vi "Test Analysis Module.vi"() -> ()   [LabVIEW 2013]
uses:
  <vilib>/rvi/Emulation/niFpgaSctlEmulationGetInTimedLoop.vi
  <vilib>/rvi/Emulation/niFpgaEmulationReportErrorSimple.vi
  <vilib>/rvi/Emulation/niFpgaGetClockAttributes.vi
  <vilib>/rvi/Emulation/niFpgaCriticalErrorInLSC.vi
  <vilib>/rvi/FIFO/Fifo_Resource/nirvififoEmulationWriteFpgaImpl.vi
  <vilib>/rvi/DataTransferAndStorage/Container/Common/niFpgaContainerGetUniqueNameForEmu.vi
  <vilib>/rvi/DataTransferAndStorage/Container/XNode/niFpgaContainer.xnode
  <vilib>/rvi/FIFO/Fifo_Resource/nirvififoEmulationWrite.vi
panel:
  in  "Acq Control.Cancel Acq":bool
  out "Accumulate Ticks":u32
  out "Analysis Ticks":u32
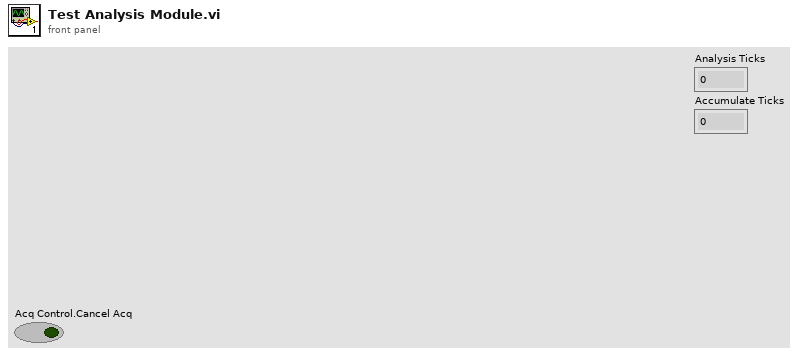
[diagram p1: front panel]
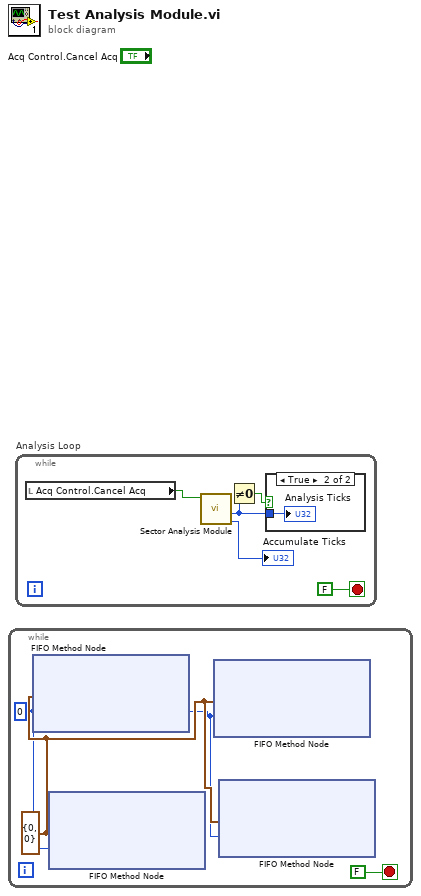
[diagram p0: block diagram]
diagram:
  n1 = while {
    stop <- FALSE stop-if-true
    w1 = 0 ("Timeout")
    w2 = cluster{"Sector #":u8, "Pixel Value":u8} {"Sector #"=0, "Pixel Value"=0} ("Element")
    n2 = xnode ("FIFO Method Node")("Element"=w2, "Timeout"=w1) -> ()  [unwired: 1 in, 2 out]
    n3 = xnode ("FIFO Method Node")("Element"=w2, "Timeout"=w1) -> ()  [unwired: 1 in, 2 out]
    n4 = xnode ("FIFO Method Node")("Element"=w2, "Timeout"=w1) -> ()  [unwired: 1 in, 2 out]
    n5 = xnode ("FIFO Method Node")("Element"=w2, "Timeout"=w1) -> ()  [unwired: 1 in, 2 out]
  }
  n6 = while "Analysis Loop" {
    stop <- FALSE stop-if-true
    n7 = local read "Acq Control.Cancel Acq"() -> (w7:bool)
    n8 = call "Sector Analysis Module.vi"("Canceled?"=w7) -> ("Accumulate Ticks"=→"Accumulate Ticks":u32, "Analysis Ticks"=w5:u32)  [unwired: 8 in, 1 out]
    n9 = Not Equal To 0?(x=w5) -> (x != 0?=w4:bool)
    n10 = case shown="True" w4 {
      tunnel: w5 -> [_ w9]
      frame False {
      }
      frame True {
        "Analysis Ticks" <- w9
      }
    }
  }
